vi "Writing to binary file.vi"(3 "error in (no error)":errorcluster, 5 "vi path":path=path "E:/Scrubbing/sceneWindowPick.vi") -> (0 "error out":errorcluster, 2 "Control Value:Get All":cluster{"Name":string, "Variant Data":variant}[](array[cluster]))   [LabVIEW 2013]
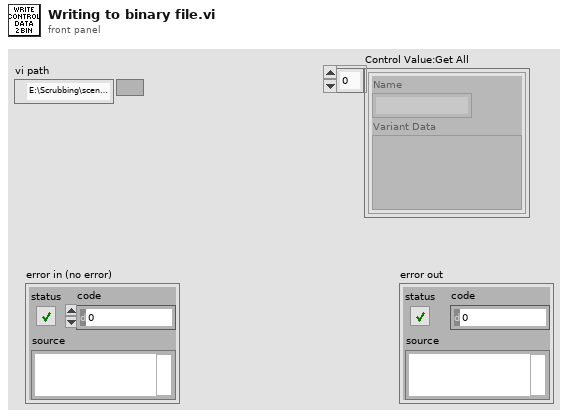
[diagram p1: front panel]
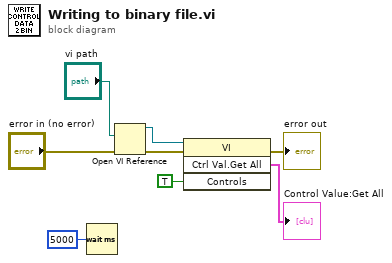
[diagram p0: block diagram]
diagram:
  n1 = Wait (ms)(milliseconds to wait=u32 5000) -> ()  [unwired: 1 out]
  n2 = Open VI Reference(vi path="vi path", error in (no error)="error in (no error)") -> (vi reference=w5:refnum<vi>, error out=w2:errorcluster)  [unwired: 4 in]
  n3 = invoke class="VI" method="Ctrl Val.Get All"(reference=w5, error in=w2, "Controls"=TRUE) -> (error out=→"error out":errorcluster, "Get All Control Values Variant"=→"Control Value:Get All":cluster{"Name":string, "Variant Data":variant}[])  [unwired: 1 in, 2 out]
